vi "Get Binning.vi"(8 "error in (no error)":errorcluster, 11 "Camera in":refnum<class "Camera.lvclass">) -> (0 "error out":errorcluster, 1 "dy":i32, 2 "dx":i32, 3 "Camera":refnum<class "Camera.lvclass">)   [LabVIEW 2020, in "Camera.lvclass"]
uses:
  Camera.lvclass
  Camera.lvclass/Camera.ctl
  Check Not Disconnected.vi
  <vilib>/Utility/error.llb/Error Cluster From Error Code.vi
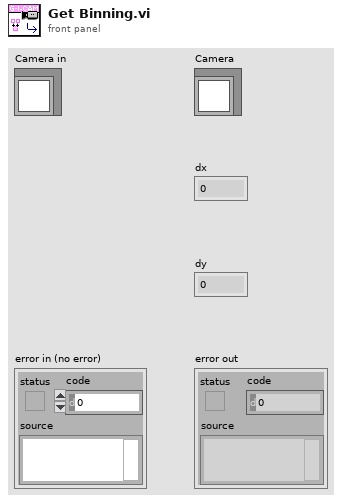
[diagram p1: front panel]
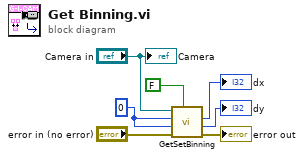
[diagram p0: block diagram]
diagram:
  w1 = 0 ("dx in")
  n1 = call "GetSetBinning.vi"("Set?"=FALSE, "error in (no error)"="error in (no error)", "dy in"=w1, "dx in"=w1, "Camera in"="Camera in") -> ("error out"=→"error out":errorcluster, "dy out"=→"dy":i32, "dx out"=→"dx":i32)  [unwired: 4 in]
  "Camera" <- "Camera in"
